vi "getExcitation.vi"(8 "error in (no error)":errorcluster, 11 "Inst.AH2500 in":refnum<class "Inst.AH2500.lvclass">) -> (0 "error out":errorcluster, 2 "Excitation (V)":dbl, 3 "Inst.AH2500 out":refnum<class "Inst.AH2500.lvclass">)   [LabVIEW 2019, in "Inst.AH2500.lvclass"]
uses:
  Inst.AH2500.lvclass
  991804cd-2d63-4689-a149-8f7b841441b7.vi
  Typedefs/Inst.AH2500.Commands--Enum.ctl
  Typedefs/Inst.AH2500.getAll--Cluster.ctl
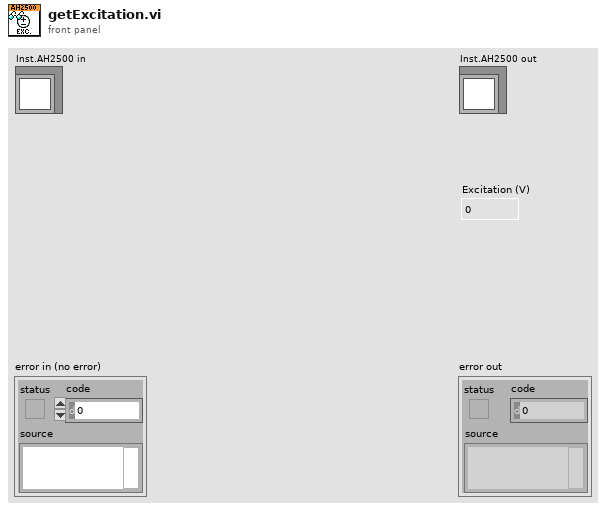
[diagram p1: front panel]
types:
  T1 = typedef "Inst.AH2500.lvclass/Inst.AH2500.getAll--Cluster.ctl" = cluster{"capacitance (pF)":dbl, "loss (nS)":dbl, "Vexc (V)":dbl}
  T2 = typedef "Inst.AH2500.lvclass/Inst.AH2500.Commands--Enum.ctl" = enum16{"getCapacitance", "getLoss", "getExcitation"}
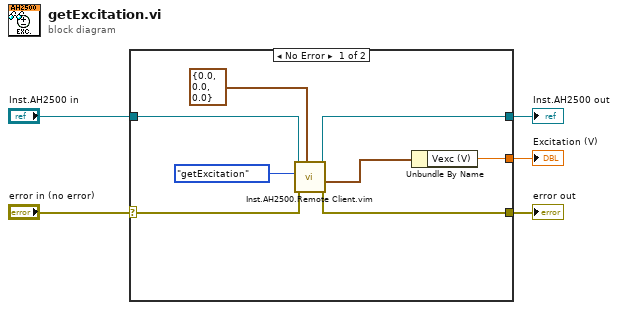
[diagram p0: block diagram]
diagram:
  n1 = case shown="No Error" "error in (no error)" {
    selector: "error in (no error)" -> [w11 w15]
    tunnel: [w10 w15] -> w4
    tunnel: [w8 w14] -> w3
    tunnel: [w13 _] -> w2
    tunnel: "Inst.AH2500 in" -> [w7 w14]
    frame No Error {
      n2 = call "Inst.AH2500.Remote Client.vim"("Data Out type"=T1 {"capacitance (pF)"=0.0, "loss (nS)"=0.0, "Vexc (V)"=0.0} ("getAll"), "error in (no error)"=w11, "Commands"=Inst.AH2500.Commands--Enum."getExcitation", "Inst.AH2500 in"=w7) -> ("error out"=w10:errorcluster, "Data out"=w9:T1, "Inst.AH2500 out"=w8:refnum<class "Inst.AH2500.lvclass">)  [unwired: 5 in]
      n3 = Unbundle By Name(w9) -> ("Vexc (V)"=w13:dbl)
    }
    frame Error {
    }
  }
  "error out" <- w4
  "Inst.AH2500 out" <- w3
  "Excitation (V)" <- w2
